vi "Read File.vi"(8 "error in (no error)":errorcluster, 11 "[Data] Userinfo Binary in":refnum<class "[Data] Userinfo Binary.lvclass">) -> (0 "error out":errorcluster, 3 "[Data] Userinfo Binary out":refnum<class "[Data] Userinfo Binary.lvclass">)   [LabVIEW 2020, in "[Data] Userinfo Binary.lvclass"]
uses:
  [Data] Userinfo Binary.lvclass
  Control/user info.ctl
  [Data] Userinfo Binary.lvclass/[Data] Userinfo Binary.ctl
  <vilib>/YU/YU-Encrypt/AES/AES.lvclass
  <vilib>/YU/YU-Encrypt/Base64/Base64.lvclass
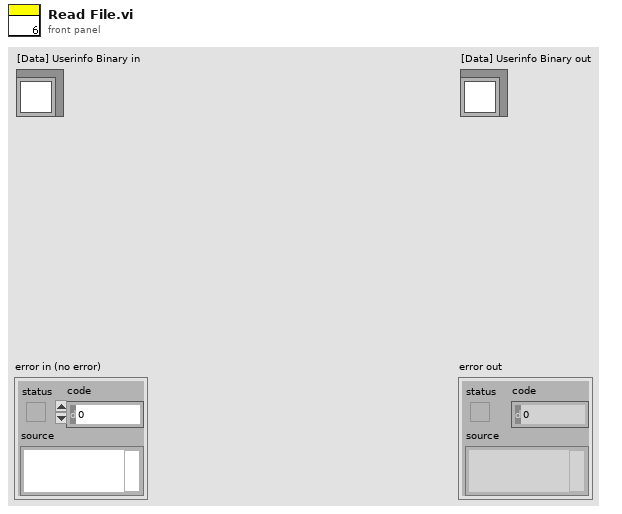
[diagram p1: front panel]
types:
  T1 = typedef "[Data] Userinfo Binary.lvclass/user info.ctl" = cluster{"password":string, "authority":i8, "department":string, "post":string, "remark":string, "create time":string, "last login time":string}
  T2 = enum16{"open", "replace", "create", "open or create", "replace or create", "replace or create with confirmation"}
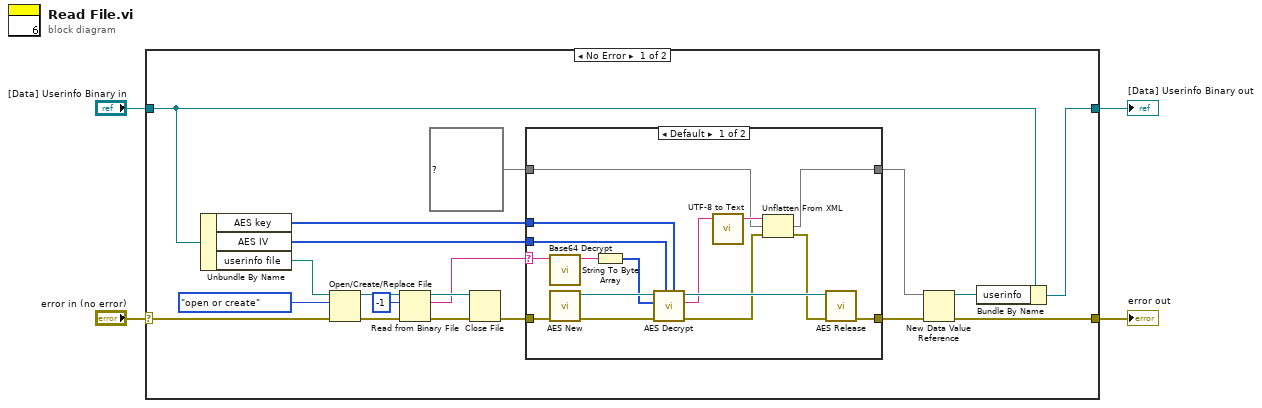
[diagram p0: block diagram]
diagram:
  n1 = case shown="No Error" "error in (no error)" {
    selector: "error in (no error)" -> [w23 w43]
    tunnel: [w9 w43] -> w3
    tunnel: [w12 w42] -> w1
    tunnel: "[Data] Userinfo Binary in" -> [w13 w42]
    frame No Error {
      n2 = Unbundle By Name(w13) -> ("AES key"=w14:u8[], "AES IV"=w15:u8[], "userinfo file"=w22:path)
      n3 = Open/Create/Replace File(file path (use dialog)=w22, error in=w23, operation (0:open)=T2."open or create") -> (refnum out=w19:refnum<file>, error out=w20:errorcluster)  [unwired: 3 in, 1 out]
      n4 = Read from Binary File(8:w20, 10:-1 ("count (1)"), 11:w19) -> (0:w18:errorcluster, 2:w5:string, 3:w17:refnum<file>)  [unwired: 3 in, 1 out]
      n5 = Close File(refnum=w17, error in=w18) -> (error out=w16:errorcluster)  [unwired: 1 out]
      n6 = case shown="Default" w5 {
        selector: w5 -> [w30 _]
        tunnel: w16 -> [w35 w41]
        tunnel: [w33 w41] -> w11
        tunnel: w15 -> [w36 _]
        tunnel: w14 -> [w37 _]
        tunnel: map{string, T1} {} ("userinfo") -> [w25 w40]
        tunnel: [w24 w40] -> w10
        frame Default {
          n7 = call <vilib>:"Base64 Decrypt.vi"("encrypted data"=w30) -> ("data"=w29:string)  [unwired: 9 in, 1 out]
          n8 = call <vilib>:"AES New.vi"("error in (no error)"=w35) -> ("error out"=w39:errorcluster, "AES out"=w38:refnum<class "AES.lvclass">)  [unwired: 9 in]
          n9 = String To Byte Array(string=w29) -> (unsigned byte array=w31:u8[])
          n10 = call <vilib>:"AES Decrypt.vi"("Key"=w37, "IV"=w36, "error in (no error)"=w39, "encrypted data"=w31, "AES in"=w38) -> ("error out"=w27:errorcluster, "data"=w32:string, "AES out"=w34:refnum<class "AES.lvclass">)  [unwired: 4 in]
          n11 = call <vilib>:"UTF-8 to Text.vi"("utf-8 text"=w32) -> ("text"=w28:string)  [unwired: 4 in]
          n12 = Unflatten From XML(xml string=w28, type=w25, error in (no error)=w27) -> (value=w24:map{string, T1}, error out=w26:errorcluster)
          n13 = call <vilib>:"AES Release.vi"("error in (no error)"=w26, "AES in"=w34) -> ("error out"=w33:errorcluster)  [unwired: 9 in]
        }
        frame "" {
        }
      }
      n14 = New Data Value Reference(data value=w10, error in=w11) -> (data value reference=w8:refnum<data-value>, error out=w9:errorcluster)
      n15 = Bundle By Name(cluster=w13, "userinfo"=w8) -> (w12:refnum<class "[Data] Userinfo Binary.lvclass">)
    }
    frame Error {
    }
  }
  "error out" <- w3
  "[Data] Userinfo Binary out" <- w1
